vi "example 9 - bool.vi"() -> ()   [LabVIEW 2020]
uses:
  ui-testing/ui-testing.lvlib
panel:
  out "Boolean":bool
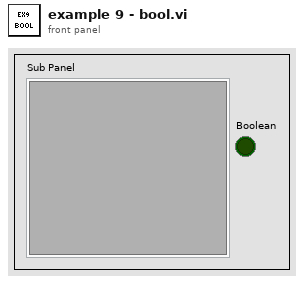
[diagram p1: front panel]
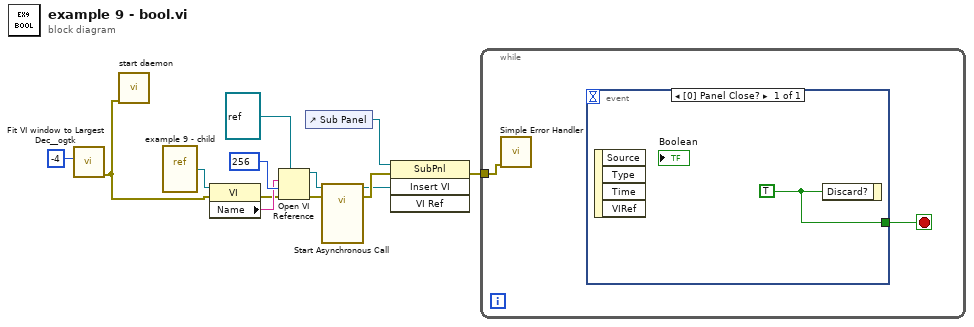
[diagram p0: block diagram]
diagram:
  n1 = call <userlib>:"Fit VI window to Largest Dec__ogtk.vi"("border spacing (2 px)"=-4) -> ("error out"=w1:errorcluster)  [unwired: 5 in, 1 out]
  n2 = call "start daemon.vi"("error in (no error)"=w1) -> ()  [unwired: 10 in, 1 out]
  n3 = vi-ref "example 9 - child.vi"() -> (w9:refnum<vi>)
  n4 = property class="VI"(reference=w9, error in=w1) -> (error out=w7:errorcluster, "Name"=w8:string)  [unwired: 1 out]
  n5 = Open VI Reference(type specifier VI Refnum (for type only)=refnum<vi> refnum, vi path=w8, options=256 ("call and forget"), error in (no error)=w7) -> (vi reference=w11:refnum<vi>, error out=w10:errorcluster)  [unwired: 2 in]
  n6 = control-ref of="Sub Panel"() -> (w3:refnum<vi>)
  n7 = call-by-ref "Start Asynchronous Call"(reference=w11, error in=w10) -> (reference out=w5:refnum<vi>, error out=w6:errorcluster)  [unwired: 12 in]
  n8 = invoke on="Invoke Node" class="SubPnl" method="Insert VI"(reference=w3, error in=w6, "VI Ref"=w5) -> (error out=w4:errorcluster)  [unwired: 1 in, 3 out]
  n9 = while {
    tunnel: w4 -> [w14]
    stop <- w15 stop-if-true
    n10 = call <vilib>:"Simple Error Handler.vi"("error in (no error)"=w14) -> ()  [unwired: 4 in, 5 out]
    n11 = event shown="[0] Panel Close?" {
      selector: _ -> [_]
      dyn-events: _ -> [_]
      timeout: _ -> [_]
      tunnel: [w16] -> w15
      event Panel Close? {
        w16 = TRUE
        n12 = event-data() -> ()  [unwired: 1 in, 4 out]
        n13 = event-data("Discard?"=w16) -> ()  [unwired: 1 in, 1 out]
      }
    }
  }
